vi "DDSTest.vi"() -> ()   [LabVIEW 2016]
panel:
  out "resulting string 4":string
  out "resulting string 3":string
  out "appended instruction string 4":string="dcp update:u\r"
  in  "phase degrees (0..360)":dbl format="%#_13g"
  in  "amplitude (0..1)":dbl=1.0 format="%#_13g"
  in  "frequency Hz (0..400M)":dbl=10000000.0 format="%#_13g"
  out "appended instruction string 2":string="dcp update:u\r"
  in  "Channels":T1(ring)=enum."Both channels"
  out "resulting string 2":string
  in  "AD9910 register name":string="STP0"
  out "single-tone profile (STP) out":u64=4611404543493626921 format="%x"
  in  "Reset string":string
  out "return count":u32=6435
  out "error out":errorcluster={"status"=TRUE, "code"=-1073807339, "source"="VISA Read in FlexDDS-NG_USB_Example.vi"}
  out "read buffer":string
  in  "FlexDDS-NG USB VISA resource name (COM)":refnum<visa-resource-name>="COM5"
  out "resulting string":string
  out "Written instruction string":string
  in  "appended instruction string":string
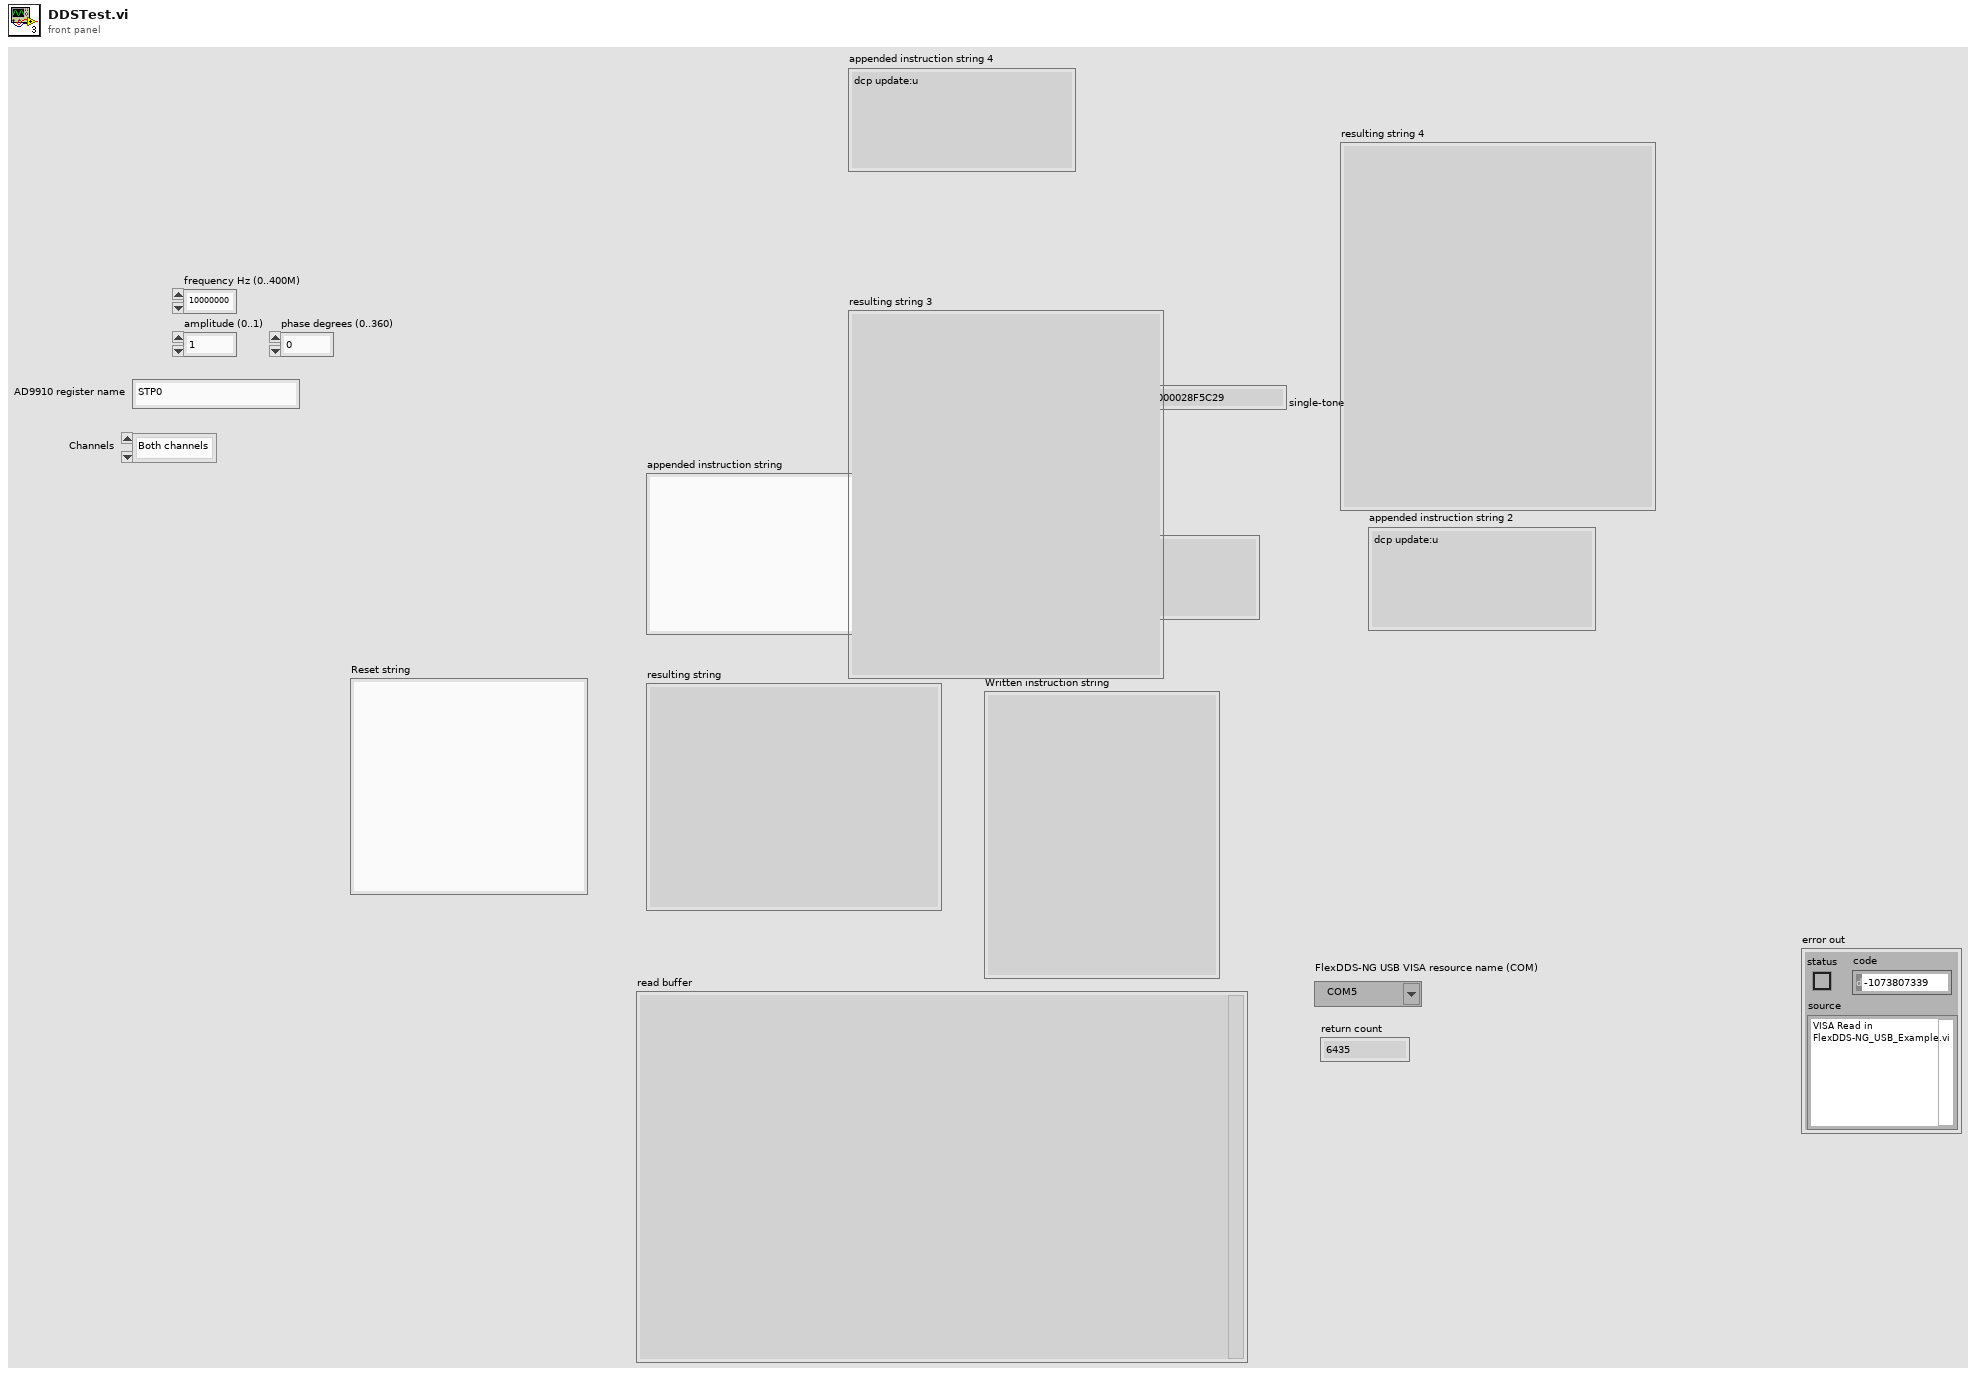
[diagram p1: front panel]
types:
  T1 = enum32{"Channel 0", "Channel 1", "Both channels"}
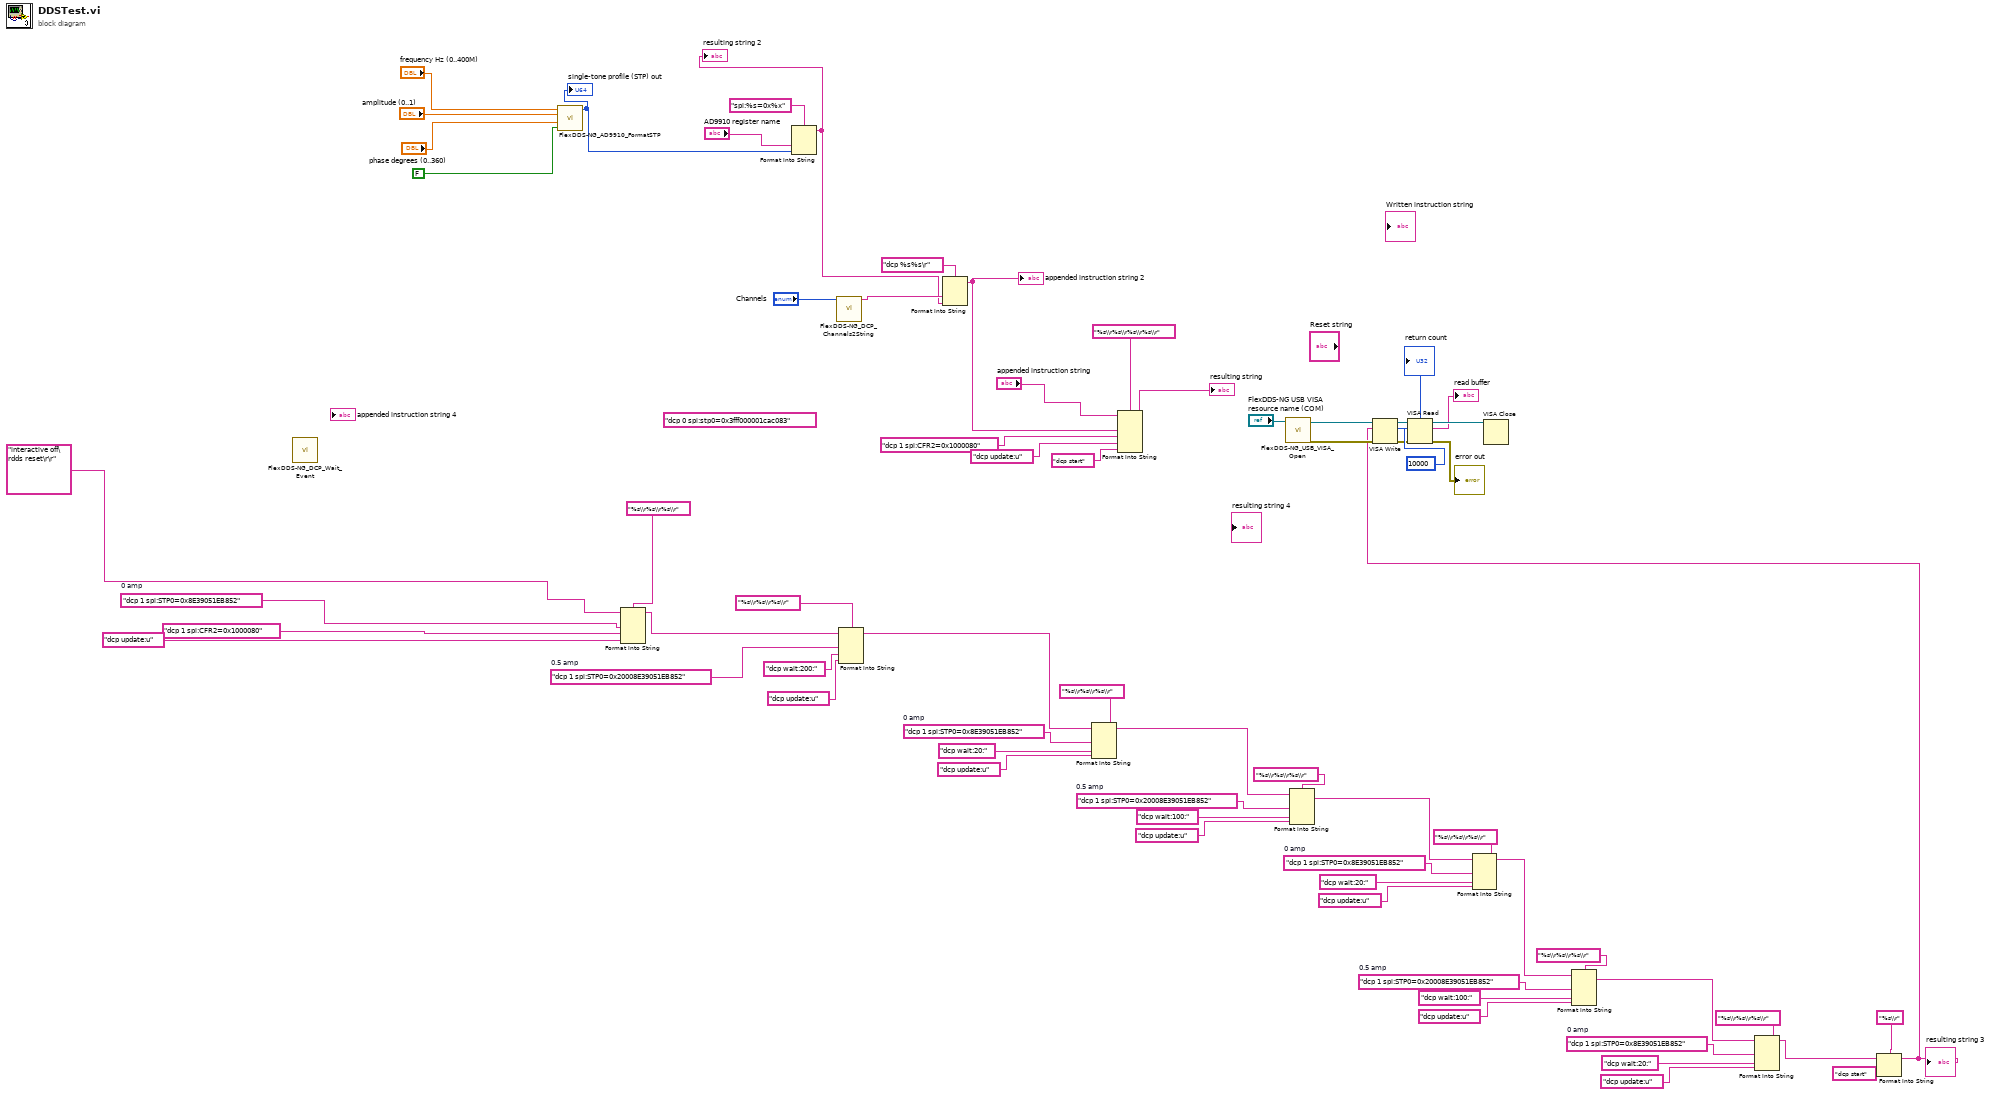
[diagram p0: block diagram]
diagram:
  w15 = "dcp 1 spi:STP0=0x8E39051EB852"  # 0 amp
  w17 = "dcp 1 spi:STP0=0x20008E39051EB852"  # 0.5 amp
  w26 = "dcp 1 spi:STP0=0x8E39051EB852"  # 0 amp
  w28 = "dcp 1 spi:STP0=0x20008E39051EB852"  # 0.5 amp
  w35 = "dcp 1 spi:STP0=0x8E39051EB852"  # 0 amp
  w7 = "dcp 1 spi:STP0=0x20008E39051EB852"  # 0.5 amp
  w37 = "dcp 1 spi:STP0=0x8E39051EB852"  # 0 amp
  (unwired) "dcp 0 spi:stp0=0x3fff000001cac083" ("input 1")
  n1 = call "FlexDDS-NG_DCP_Wait_Event.vi"() -> ()  [unwired: 11 in, 1 out]
  n2 = call "FlexDDS-NG_AD9910_FormatSTP.vi"("mirror frequency?"=FALSE, "phase degrees (0..360)"="phase degrees (0..360)", "amplitude (0..1)"="amplitude (0..1)", "frequency Hz (0..400M)"="frequency Hz (0..400M)") -> ("single-tone profile (STP) out"=w49:u64)  [unwired: 4 in, 3 out]
  "single-tone profile (STP) out" <- w49
  n3 = Format Into String(format string="%s\\r%s\\r%s\\r", initial string="interactive off\rdds reset\r\r" ("appended instruction string 5"), w37, "dcp 1 spi:CFR2=0x1000080", "dcp update:u" ("input 2")) -> (resulting string=w4:string)  [unwired: 1 in, 1 out]
  n4 = Format Into String(format string="spi:%s=0x%x", "AD9910 register name", w49) -> (resulting string=w45:string)  [unwired: 2 in, 1 out]
  "resulting string 2" <- w45
  n5 = call "FlexDDS-NG_DCP_Channels2String.vi"("Channels"="Channels") -> ("channels string"=w46:string)  [unwired: 10 in]
  n6 = Format Into String(format string="%s\\r%s\\r%s\\r", initial string=w4, w7, "dcp wait:200:", "dcp update:u" ("input 2")) -> (resulting string=w3:string)  [unwired: 1 in, 1 out]
  n7 = Format Into String(format string="dcp %s%s\r", w46, w45) -> (resulting string=w36:string)  [unwired: 2 in, 1 out]
  "appended instruction string 2" <- w36
  n8 = Format Into String(format string="%s\\r%s\\r%s\\r", initial string=w3, w35, "dcp wait:20:", "dcp update:u" ("input 2")) -> (resulting string=w29:string)  [unwired: 1 in, 1 out]
  n9 = Format Into String(format string="%s\\r%s\\r%s\\r%s\\r", initial string="appended instruction string", w36, "dcp 1 spi:CFR2=0x1000080", "dcp update:u" ("input 2"), "dcp start" ("input 4")) -> (resulting string=→"resulting string":string)  [unwired: 1 in, 1 out]
  n10 = call "FlexDDS-NG_USB_VISA_Open.vi"("FlexDDS-NG USB VISA resource name (COM)"="FlexDDS-NG USB VISA resource name (COM)") -> ("error out"=w65:errorcluster, "FlexDDS-NG USB VISA resource name out"=w66:refnum<visa-resource-name>)  [unwired: 9 in]
  n11 = Format Into String(format string="%s\\r%s\\r%s\\r", initial string=w29, w28, "dcp wait:100:", "dcp update:u" ("input 2")) -> (resulting string=w23:string)  [unwired: 1 in, 1 out]
  n12 = Format Into String(format string="%s\\r%s\\r%s\\r", initial string=w23, w26, "dcp wait:20:", "dcp update:u" ("input 2")) -> (resulting string=w10:string)  [unwired: 1 in, 1 out]
  n13 = Format Into String(format string="%s\\r%s\\r%s\\r", initial string=w10, w17, "dcp wait:100:", "dcp update:u" ("input 2")) -> (resulting string=w12:string)  [unwired: 1 in, 1 out]
  n14 = Format Into String(format string="%s\\r%s\\r%s\\r", initial string=w12, w15, "dcp wait:20:", "dcp update:u" ("input 2")) -> (resulting string=w9:string)  [unwired: 1 in, 1 out]
  n15 = Format Into String(format string="%s\\r", initial string=w9, "dcp start" ("input 4")) -> (resulting string=w8:string)  [unwired: 1 in, 1 out]
  "resulting string 3" <- w8
  n16 = VISA Write(VISA resource name=w66, write buffer=w8, error in (no error)=w65) -> (VISA resource name out=w61:refnum<visa-resource-name>, return count=→"return count":u32, error out=w59:errorcluster)
  n17 = VISA Read(VISA resource name=w61, byte count=u32 10000, error in (no error)=w59) -> (VISA resource name out=w64:refnum<visa-resource-name>, read buffer=→"read buffer":string, error out=→"error out":errorcluster)  [unwired: 1 out]
  n18 = VISA Close(VISA resource name=w64) -> ()  [unwired: 1 in, 1 out]
